vi "setUp.vi"(8 "error in (no error)":errorcluster, 11 "reference in":refnum<class "Read Section - Path Tests.lvclass">) -> (0 "error out":errorcluster, 3 "reference out":refnum<class "Read Section - Path Tests.lvclass">)   [LabVIEW 2017, in "Read Section - Path Tests.lvclass"]
doc: "setUp runs prior to the test method during test execution. Use this method to initialize any object data required by your tests."
uses:
  Read Section - Path Tests.lvclass
  Read File Tests.lvclass
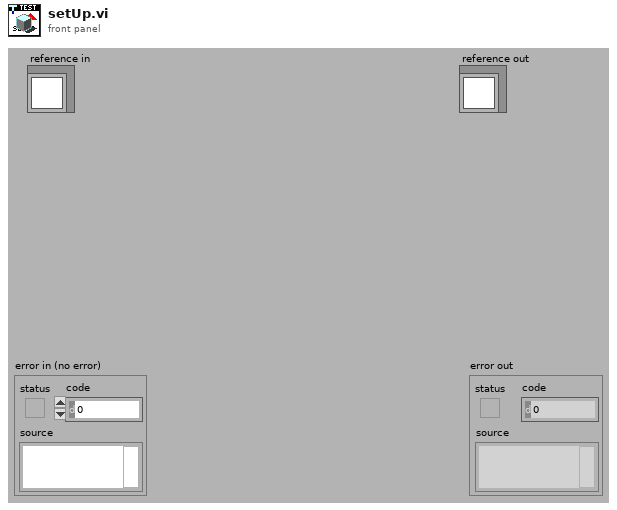
[diagram p1: front panel]
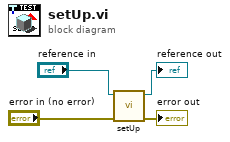
[diagram p0: block diagram]
diagram:
  n1 = call-parent "setUp.vi"("error in (no error)"="error in (no error)", "reference in"="reference in") -> ("error out"=→"error out":errorcluster, "reference out"=→"reference out":refnum<class "Read Section - Path Tests.lvclass">)  [unwired: 8 in]
